vi "Benchmark Running.vi"(8 "error in (no error)":errorcluster, 11 "CIFCorePlugin in":refnum<class "CIFCorePlugin.lvclass">) -> (0 "error out":errorcluster, 3 "CIFCorePlugin out":refnum<class "CIFCorePlugin.lvclass">)   [LabVIEW 2021, in "CIFCorePlugin.lvclass"]
uses:
  CIFCorePlugin.lvclass
  CIFCorePlugin.lvclass/CIFCorePlugin.ctl
  Accessors/Get Time.vi
  Accessors/Timestamps/Read Execute TS.vi
  Accessors/Timestamps/Read Housekeeping TS.vi
  Accessors/Timestamps/Read Sleep TS.vi
  Accessors/Timestamps/Read Target Wake TS.vi
  CIFUtilities/CIFClocks/SubVIs/Add Error.vi
  CIFUtilities/CIFClocks/Core/Get Time.vi
  Common/Utilities/Append Error Location.vi
  CIFUtilities/CIFClocks/Time Conversion/LabVIEW Time to UTC Time.vi
  Common/CIFCoreCommon.lvlib
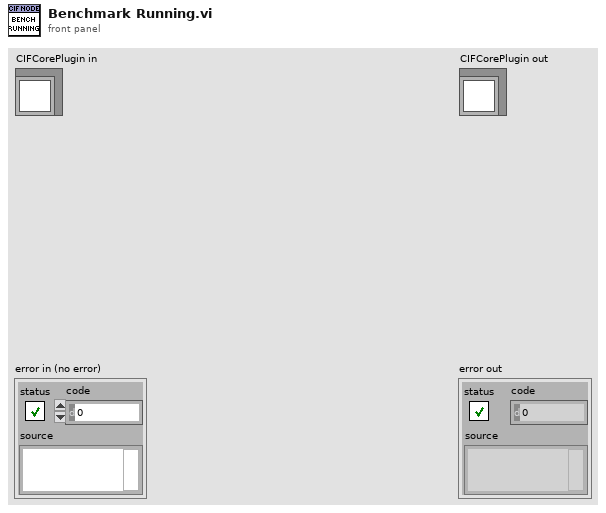
[diagram p1: front panel]
types:
  T1 = typedef "CIFCoreCommon.lvlib/Timing Stats Base.ctl" = cluster{"Max":i32, "Min":i32}
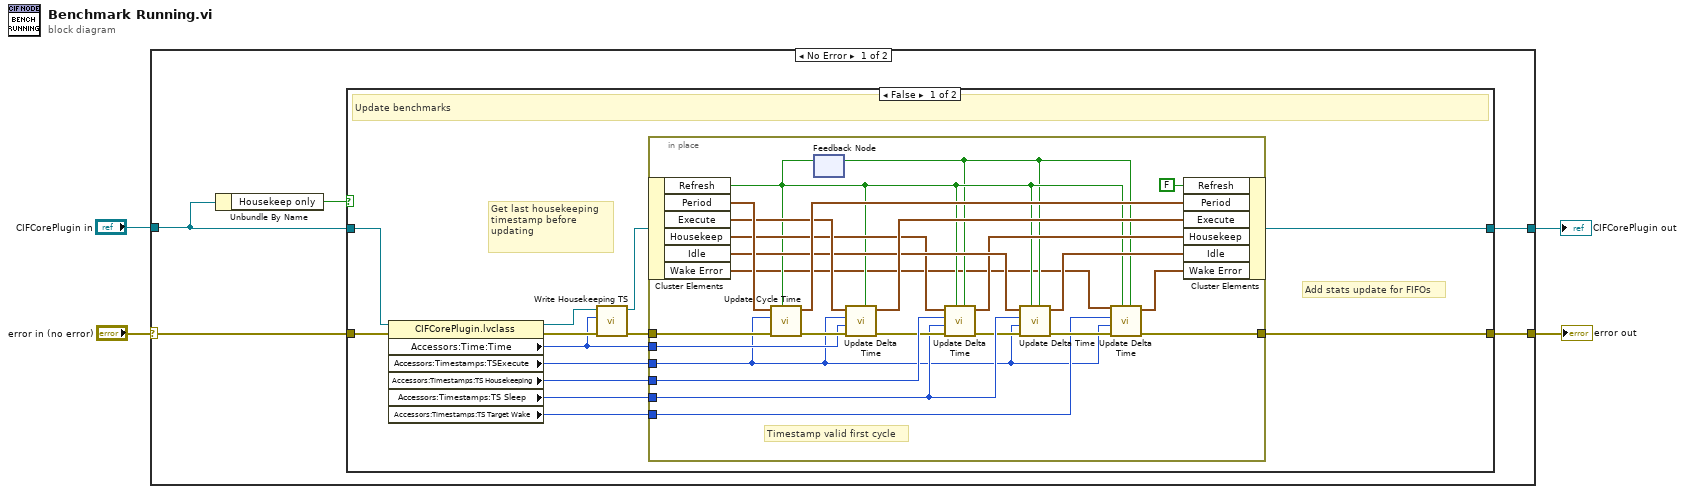
[diagram p0: block diagram]
diagram:
  n1 = case shown="No Error" "error in (no error)" {
    selector: "error in (no error)" -> [w9 w50]
    tunnel: [w7 w50] -> w1
    tunnel: [w8 w49] -> w2
    tunnel: "CIFCorePlugin in" -> [w6 w49]
    frame No Error {
      n2 = Unbundle By Name(w6) -> ("Housekeep only"=w5:bool)
      n3 = case shown="False" w5 {
        tunnel: w9 -> [w22 w47]
        tunnel: [w13 w48] -> w8
        tunnel: [w12 w47] -> w7
        tunnel: w6 -> [w10 w48]
        frame False {
          # "Get last housekeeping timestamp before updating"
          # "Add stats update for FIFOs"
          # "Update benchmarks"
          n4 = property class="CIFCorePlugin.lvclass"(reference=w10, error in=w22) -> (reference out=w16:refnum<class "CIFCorePlugin.lvclass">, error out=w18:errorcluster, "Accessors:Time:Time"=w14:u64, "Accessors:Timestamps:TSExecute"=w19:u64, "Accessors:Timestamps:TS Housekeeping"=w20:u64, "Accessors:Timestamps:TS Sleep"=w21:u64, "Accessors:Timestamps:TS Target Wake"=w11:u64)
          n5 = call "Write Housekeeping TS.vi"("error in (no error)"=w18, "Housekeeping"=w14, "CIFCorePlugin in"=w16) -> ("error out"=w17:errorcluster, "CIFCorePlugin out"=w15:refnum<class "CIFCorePlugin.lvclass">)  [unwired: 7 in]
          n6 = in-place {
            in-place-border: w19 -> [w23]
            in-place-border: w20 -> [w39]
            in-place-border: w21 -> [w37]
            in-place-border: w17 -> [w43]
            in-place-border: [w29] -> w12
            in-place-border: w14 -> [w31]
            in-place-border: w11 -> [w24]
            # "Timestamp valid first cycle"
            n7 = in-place-cluster #1(w15) -> ("Refresh"=w28:bool, "Period"=w46:T1, "Execute"=w41:T1, "Housekeep"=w35:T1, "Idle"=w36:T1, "Wake Error"=w26:T1)
            n8 = call "Update Cycle Time.vi"("Initialize"=w28, "error in (no error)"=w43, "T1"=w23, "Timing in"=w46) -> ("error out"=w42:errorcluster, "Timing out"=w44:cluster{"Max":i32, "Min":i32})  [unwired: 6 in]
            n9 = feedback-in #2(w28) -> ()
            n10 = feedback #2() -> (w27:bool)  [unwired: 1 in]
            n11 = call "Update Delta Time.vi"("reinit"=w28, "error in (no error)"=w42, "T2"=w31, "T1"=w23, "Timing in"=w41) -> ("error out"=w38:errorcluster, "Timing out"=w40:cluster{"Max":i32, "Min":i32})  [unwired: 5 in]
            n12 = call "Update Delta Time.vi"("reinit"=w27, "skip"=w28, "error in (no error)"=w38, "T2"=w37, "T1"=w39, "Timing in"=w35) -> ("error out"=w32:errorcluster, "Timing out"=w33:cluster{"Max":i32, "Min":i32})  [unwired: 4 in]
            n13 = call "Update Delta Time.vi"("reinit"=w27, "skip"=w28, "error in (no error)"=w32, "T2"=w23, "T1"=w37, "Timing in"=w36) -> ("error out"=w30:errorcluster, "Timing out"=w34:cluster{"Max":i32, "Min":i32})  [unwired: 4 in]
            n14 = call "Update Delta Time.vi"("reinit"=w27, "skip"=w28, "error in (no error)"=w30, "T2"=w23, "T1"=w24, "Timing in"=w26) -> ("error out"=w29:errorcluster, "Timing out"=w25:cluster{"Max":i32, "Min":i32})  [unwired: 4 in]
            n15 = in-place-cluster #1("Refresh"=FALSE, "Period"=w44, "Execute"=w40, "Housekeep"=w33, "Idle"=w34, "Wake Error"=w25) -> (w13:refnum<class "CIFCorePlugin.lvclass">)
          }
        }
        frame True {
          # "Housekeep only.  Don't update benchmarks since execute never ran."
        }
      }
    }
    frame Error {
    }
  }
  "error out" <- w1
  "CIFCorePlugin out" <- w2
